vi "Test Copy Raw Memory To Image ARGB.vi"(8 "error in (no error)":errorcluster, 11 "Test Case In":refnum<class "Image.lvclass">) -> (0 "error out":errorcluster, 3 "Test Case Out":refnum<class "Image.lvclass">)   [LabVIEW 2020, in "g_ar_toolkit.test.lvlib" / "Image.lvclass"]
uses:
  Image.lvclass
  C:/Program Files (x86)/National Instruments/LabVIEW 2020/vi.lib/Astemes/LUnit/Test Case.lvclass
  g_ar_toolkit.common/Image Size (Integer).ctl
  g_ar_toolkit.image/Raw Memory Information.ctl
  g_ar_toolkit.image/Raw Memory Information Dimension.ctl
  <vilib>/Astemes/LUnit/Test Case.lvclass/Test Case.ctl
  g_ar_toolkit.image/CreateEmptyImageARGB.vi
  4993e8ee-a06a-463a-9684-69129f64d5ce.vi
  g_ar_toolkit.image/Copy Array to Image.vi
  g_ar_toolkit.image/CopyArrayToImageARGB.vi
  g_ar_toolkit.image/CreateEmptyImageARGB.vi/3321fa97-f432-4e1e-8db9-a0df79aed21b.vi
  g_ar_toolkit.image/CopyRawMemoryToImageARGB.vi/e0109ec8-11ee-4a07-aeee-d632e4e22c38.vi
  <vilib>/Astemes/LUnit/Append Pass Result.vi
  <vilib>/Astemes/LUnit/Append Fail Result.vi
  <vilib>/Astemes/LUnit/Describe Comparison.vi
  <vilib>/Astemes/LUnit/Compare Variants.vi
  g_ar_toolkit.image/CopyArrayToImageARGB.vi/26c70cee-9332-41f4-9755-08948a885cbe.vi
  <vilib>/Astemes/LUnit/Run In UI.vi
  <vilib>/Utility/error.llb/Clear Errors.vi
  g_ar_toolkit.image/ARGBColourToU32.vi
  g_ar_toolkit.common/Module Path.vi
  <vilib>/Utility/error.llb/Error Cluster From Error Code.vi
  <vilib>/picture/pixmap.llb/Flatten Pixmap.vi
  <vilib>/Astemes/LUnit/Describe Variant.vi
  Image.lvclass/Image.ctl
  g_ar_toolkit.image/g_ar_toolkit.image.lvlib
  g_ar_toolkit.common/g_ar_toolkit.common.lvlib
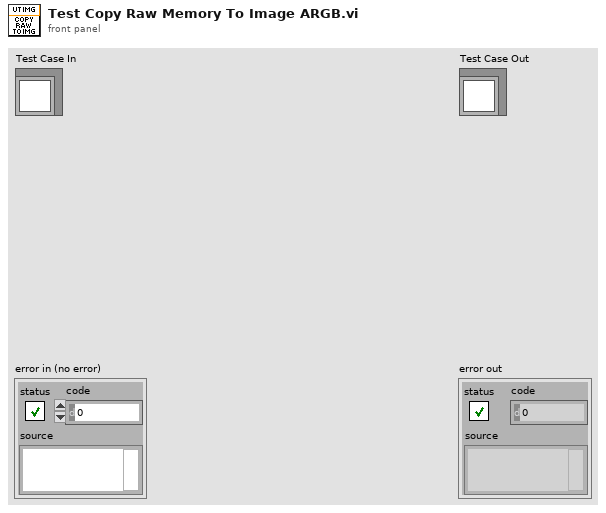
[diagram p1: front panel]
types:
  T1 = typedef "g_ar_toolkit.common.lvlib/Image Size (Integer).ctl" = cluster{"Width":u16, "Height":u16}
  T2 = typedef "g_ar_toolkit.image.lvlib/Raw Memory Information.ctl" = cluster{"Memory Address":u64, "Dimension 0":T3, "Dimension 1":T3}
  T3 = typedef "g_ar_toolkit.image.lvlib/Raw Memory Information Dimension.ctl" = cluster{"Size":u16, "Stride":u32}
  T4 = cluster{"pointer":u64, "size_0":u32, "stride_0":i32, "size_1":u32, "stride_1":i32, "element size":u32, "subarray?":bool}
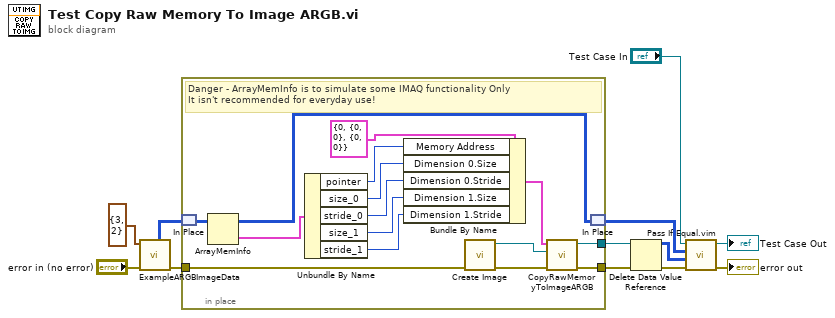
[diagram p0: block diagram]
diagram:
  n1 = call "ExampleARGBImageData.vi"("error in (no error)"="error in (no error)", "Image Size"=T1 {"Width"=3, "Height"=2}) -> ("error out"=w2:errorcluster, "ARGB Array Data"=w4:u32[][])  [unwired: 6 in, 2 out]
  n2 = in-place "In Place Element Structure" {
    in-place-border: [w18] -> w9
    in-place-border: w2 -> [w16]
    in-place-border: [w15] -> w7
    # "Danger - ArrayMemInfo is to simulate some IMAQ functionality Only\nIt isn't recommended for everyday use!"
    n3 = in-place-match #1(w4) -> (w14:u32[][])
    n4 = ArrayMemInfo(3:w14) -> (0:w27:T4, 1:w13:u32[][])
    n5 = Unbundle By Name(w27) -> ("pointer"=w26:u64, "size_0"=w24:u32, "stride_0"=w23:i32, "size_1"=w21:u32, "stride_1"=w22:i32)
    n6 = Bundle By Name(cluster=T2 {"Memory Address"=0, "Dimension 0"={"Size"=0, "Stride"=0}, "Dimension 1"={"Size"=0, "Stride"=0}} ("Source"), "Memory Address"=w26, "Dimension 0.Size"=w24, "Dimension 0.Stride"=w23, "Dimension 1.Size"=w21, "Dimension 1.Stride"=w22) -> (w19:T2)
    n7 = call-poly "Create Image.vi"("error in (no error)"=w16) -> ("error out"=w17:errorcluster, "New ARGB Image"=w25:refnum<data-value>)  [unwired: 9 in]
    n8 = call "CopyRawMemoryToImageARGB.vi"("error in (no error)"=w17, "ARGB Image Destination"=w25, "Source"=w19) -> ("error out"=w15:errorcluster, "ARGB Image Destination (Duplicate)"=w18:refnum<data-value>)  [unwired: 7 in]
    n9 = in-place-match #1(w13) -> (w5:u32[][])
  }
  n10 = Delete Data Value Reference(data value reference=w9, error in=w7) -> (data value=w8:u32[][], error out=w6:errorcluster)
  n11 = call "Pass If Equal.vim"("error in (no error)"=w6, "Actual"=w8, "Expected"=w5, "LUnit Test Case In"="Test Case In") -> ("error out"=→"error out":errorcluster, "LUnit Test Case Out"=→"Test Case Out":refnum<class "Image.lvclass">)  [unwired: 6 in]
